vi "pbw_calc_connect.vi"(3 "error in":errorcluster, 4 "identity":string="bias", 5 "ctx in":T1 format="%.0x") -> (0 "error out":errorcluster, 2 "socket out":T1 format="%.0x")   [LabVIEW 2010]
uses:
  <vilib>/addons/zeromq/pointer.ctl
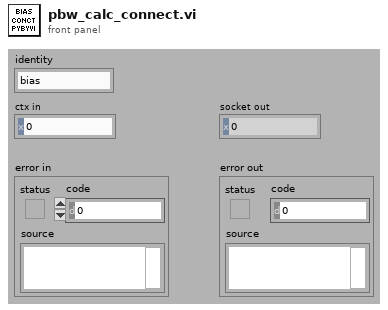
[diagram p1: front panel]
types:
  T1 = typedef "pointer.ctl" = u64
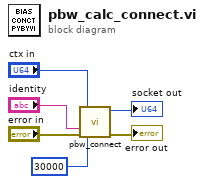
[diagram p0: block diagram]
diagram:
  n1 = call <vilib>:"pbw_connect.vi"("error in"="error in", "identity"="identity", "startup delay (ms)"=u32 30000, "ctx in"="ctx in") -> ("error out"=→"error out":errorcluster, "socket out"=→"socket out":T1)  [unwired: 2 in]
